vi "register update callback.vi"(8 "error in":errorcluster, 9 "controls":refnum<vi>[](array[refnum]), 10 "VI Refnum":refnum<vi>, 11 "displayable in":refnum<class "displayable.lvclass">) -> (0 "error out":errorcluster, 3 "displayable out":refnum<class "displayable.lvclass">)   [LabVIEW 2013, in "displayable.lvclass"]
uses:
  displayable.lvclass
  displayable.lvclass/displayable.ctl
  callback settings.ctl
  <vilib>/Utility/VariantDataType/VariantType.lvlib
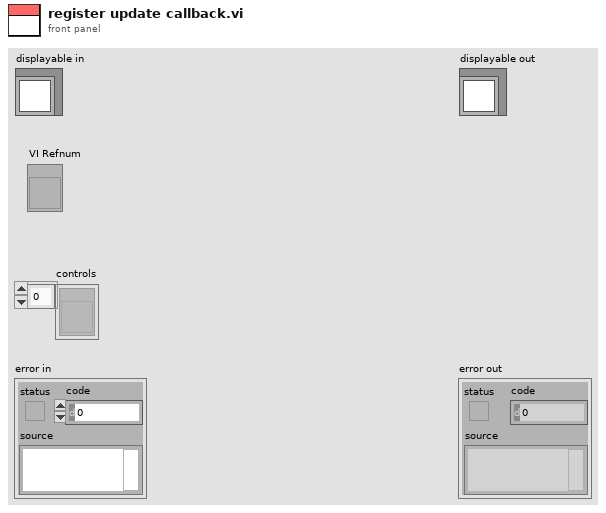
[diagram p1: front panel]
types:
  T1 = typedef "displayable.lvclass/callback settings.ctl" = cluster{"VI Refnum":refnum<vi>, "displayable":refnum<data-value>, "oi":string, "oo":string, "di":string}
  T2 = typedef "VariantType.lvlib/Type.ctl" = enum8{"Invalid Type", "Void", "I8", "I16", "I32", "I64", "U8", "U16", "U32", "U64", "Single Float", "Double Float", "Extended Float", "Single Complex", "Double Complex", "Extended Complex", "Enum U8", "Enum U16", "Enum U32", "Enum U64", "Single Float With Unit", "Double Float With Unit", "Extended Float With Unit", "Single Complex with Unit", "Double Complex with Unit", "Extended Complex with Unit", "Boolean", "String", "Path", "Picture", "Tag", "Array", "Cluster", "Variant", "LV Variant", "Waveform", "Timestamp", "Digital Waveform", "Digital Data", "ExpressData", "Refnum", "External Data", "VI", "Poly VI", "LabVIEW Class Instance", "Fixed Point"}
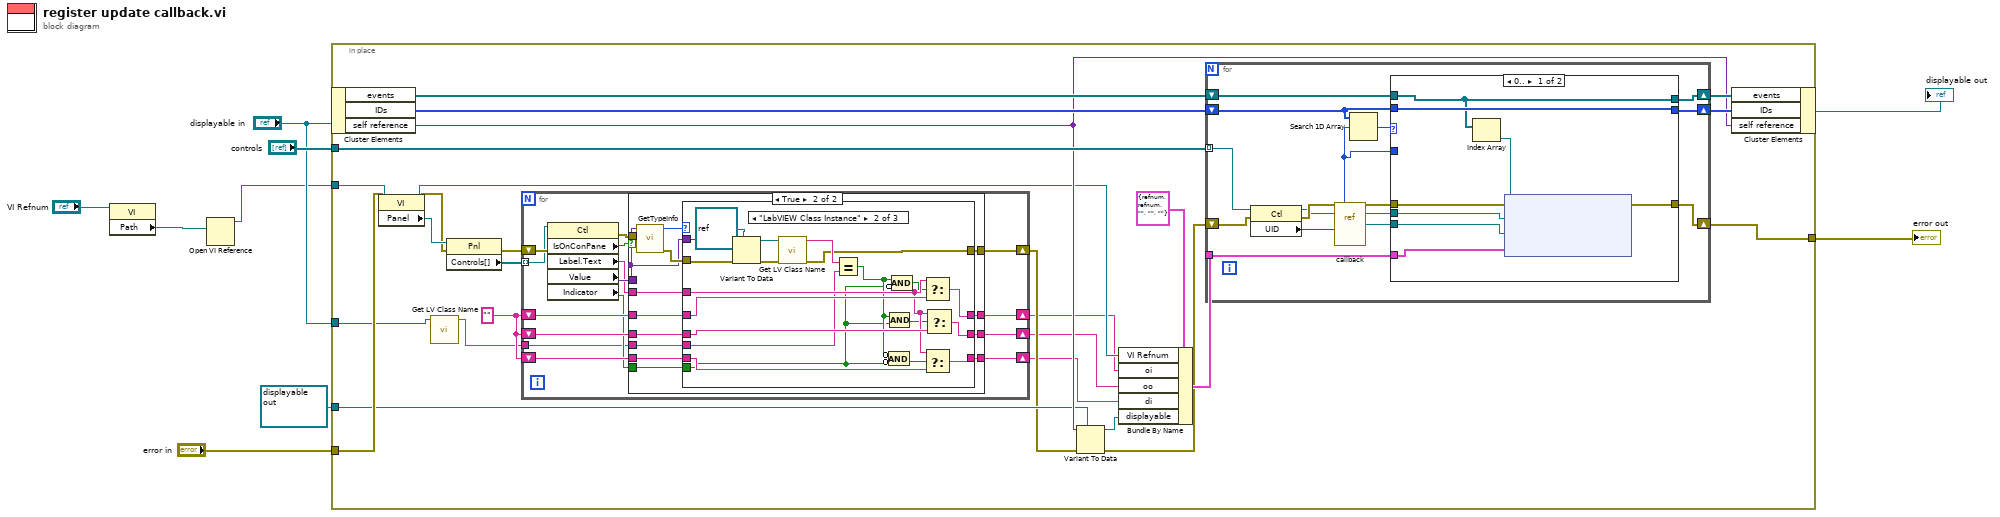
[diagram p0: block diagram]
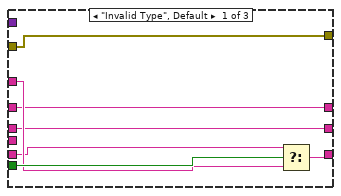
[diagram p3: hidden frame]
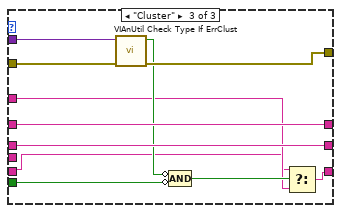
[diagram p4: hidden frame]
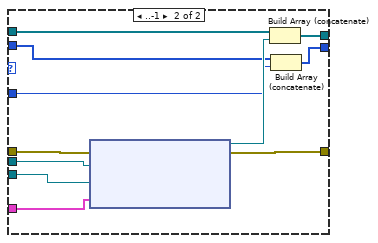
[diagram p5: hidden frame]
diagram:
  n1 = property class="VI"(reference="VI Refnum") -> ("Path"=w2:path)  [unwired: 1 in, 2 out]
  n2 = Open VI Reference(vi path=w2) -> (vi reference=w1:refnum<vi>)  [unwired: 5 in, 1 out]
  n3 = in-place {
    in-place-border: "controls" -> [w35]
    in-place-border: "error in" -> [w23]
    in-place-border: [w30] -> w6
    in-place-border: w1 -> [w27]
    in-place-border: refnum<data-value> refnum ("displayable") -> [w19]
    in-place-border: "displayable in" -> [w11]
    w15 = ""
    n4 = in-place-cluster #1("displayable in") -> ("events"=w34:refnum<k27>[], "IDs"=w33:i32[], "self reference"=w25:variant)
    n5 = property class="VI"(reference=w27, error in=w23) -> (reference out=w24:refnum<vi>, error out=w21:errorcluster, "Panel"=w22:refnum<vi>)
    n6 = call <vilib>:"Get LV Class Name.vi"("object"=w11) -> ("class name"=w10:string)  [unwired: 9 in, 1 out]
    n7 = property class="Pnl"(reference=w22, error in=w21) -> (error out=w17:errorcluster, "Controls[]"=w18:refnum<vi>[])  [unwired: 1 out]
    n8 = for {
      tunnel: w18 -> [w49] mode=indexing
      shift-right: [w46] -> w16
      shift-left: w17 -> [w50]
      shift-right: [w43] -> w14
      shift-left: w15 -> [w44]
      shift-right: [w42] -> w12
      shift-left: w15 -> [w41]
      shift-right: [w39] -> w13
      shift-left: w15 -> [w40]
      tunnel: w10 -> [w36]
      n9 = property class="Ctl"(reference=w49, error in=w50) -> (error out=w48:errorcluster, "IsOnConPane"=w45:bool, "Label.Text"=w37:string, "Value"=w47:variant, "Indicator"=w38:bool)  [unwired: 1 out]
      n10 = case shown="True" w45 {
        tunnel: w48 -> [w54 w68]
        tunnel: w47 -> [_ w65]
        tunnel: [w54 w64] -> w46
        tunnel: w44 -> [w53 w62]
        tunnel: [w53 w63] -> w43
        tunnel: [w52 w61] -> w42
        tunnel: w41 -> [w52 w60]
        tunnel: w40 -> [w51 w59]
        tunnel: [w51 w56] -> w39
        tunnel: w38 -> [_ w58]
        tunnel: w37 -> [_ w57]
        tunnel: w36 -> [_ w55]
        frame False {
        }
        frame True {
          n11 = call <vilib>:"GetTypeInfo.vi"("error in (no error)"=w68, "Variant"=w65) -> ("error out"=w66:errorcluster, "Type Enum"=w67:T2)  [unwired: 5 in, 3 out]
          n12 = case shown="\"LabVIEW Class Instance\"" w67 {
            tunnel: w66 -> [w69 w82 w106]
            tunnel: w65 -> [_ w81 w105]
            tunnel: [w69 w77 w104] -> w64
            tunnel: [w70 w95 w103] -> w63
            tunnel: w62 -> [w70 w90 w103]
            tunnel: [w71 w93 w102] -> w61
            tunnel: w60 -> [w71 w91 w102]
            tunnel: w59 -> [w73 w92 w97]
            tunnel: w58 -> [w75 w83 w100]
            tunnel: w57 -> [w74 w89 w98]
            tunnel: [w72 w94 w96] -> w56
            tunnel: w55 -> [_ w88 _]
            frame "Invalid Type", Default {
              n13 = Select(t=w73, s=w75, f=w74) -> (s? t:f=w72:string)
            }
            frame "LabVIEW Class Instance" {
              n14 = Variant To Data(error in=w82, type=refnum<class> refnum ("LabVIEW Object"), Variant=w81) -> (data=w79:refnum<class>, error out=w80:errorcluster)
              n15 = call <vilib>:"Get LV Class Name.vi"("error in (no error)"=w80, "object"=w79) -> ("error out"=w77:errorcluster, "class name"=w78:string)  [unwired: 8 in]
              n16 = Equal?(x=w78, y=w88) -> (x = y?=w84:bool)
              n17 = Compound Arithmetic op=AND(invert w84, invert w83) -> (w85:bool)
              n18 = Compound Arithmetic op=AND(w84, w83) -> (w87:bool)
              n19 = Compound Arithmetic op=AND(w84, invert w83) -> (w86:bool)
              n20 = Select(t=w89, s=w86, f=w90) -> (s? t:f=w95:string)
              n21 = Select(t=w89, s=w85, f=w92) -> (s? t:f=w94:string)
              n22 = Select(t=w89, s=w87, f=w91) -> (s? t:f=w93:string)
            }
            frame "Cluster" {
              n23 = call <vilib>:"VIAnUtil Check Type If ErrClust.vi"("error in (no error)"=w106, "Data In"=w105) -> ("error out"=w104:errorcluster, "IsErrClust?"=w101:bool)  [unwired: 8 out]
              n24 = Compound Arithmetic op=AND(invert w101, invert w100) -> (w99:bool)
              n25 = Select(t=w97, s=w99, f=w98) -> (s? t:f=w96:string)
            }
          }
        }
      }
    }
    n26 = Variant To Data(error in=w16, type=w19, Variant=w25) -> (data=w20:refnum<data-value>, error out=w26:errorcluster)
    n27 = Bundle By Name(cluster=T1 {"VI Refnum"=refnum, "displayable"=refnum, "oi"="", "oo"="", "di"=""} ("callback settings"), "VI Refnum"=w24, "oi"=w14, "oo"=w12, "di"=w13, "displayable"=w20) -> (w28:T1)
    n28 = for {
      tunnel: w35 -> [w119] mode=indexing
      shift-right: [w113] -> w31
      shift-left: w33 -> [w111]
      shift-right: [w112] -> w32
      shift-left: w34 -> [w114]
      shift-right: [w116] -> w30
      shift-left: w26 -> [w118]
      tunnel: w28 -> [w108]
      n29 = property class="Ctl"(reference=w119, error in=w118) -> (reference out=w109:refnum<vi>, error out=w117:errorcluster, "UID"=w110:i32)
      n30 = vi-ref "callback.vi"() -> ("vi reference"=w107:refnum<vi>)
      n31 = Search 1D Array(1D array=w111, element=w110) -> (index of element=w115:i32)  [unwired: 1 in]
      n32 = case shown="0.." w115 {
        tunnel: w117 -> [w125 w138]
        tunnel: [w123 w137] -> w116
        tunnel: w114 -> [w126 w136]
        tunnel: [w127 w134] -> w113
        tunnel: [w126 w133] -> w112
        tunnel: w111 -> [w127 w132]
        tunnel: w110 -> [_ w131]
        tunnel: w109 -> [w121 w130]
        tunnel: w108 -> [w120 w129]
        tunnel: w107 -> [w122 w128]
        frame 0.. {
          n33 = Index Array(array=w126) -> (element=w124:refnum<k27>)  [unwired: 1 in]
          n34 = node(w124, w125, w121, w122, w120) -> (w123:errorcluster)  [unwired: 1 out]
        }
        frame ..-1 {
          n35 = node(w138, w130, w128, w129) -> (w135:refnum<k27>, w137:errorcluster)  [unwired: 1 in]
          n36 = Build Array (concatenate)(w136, w135) -> (w133:refnum<k27>[])
          n37 = Build Array (concatenate)(w132, w131) -> (w134:i32[])
        }
      }
    }
    n38 = in-place-cluster #1("events"=w32, "IDs"=w31, "self reference"=w25) -> (→"displayable out":refnum<class "displayable.lvclass">)
  }
  "error out" <- w6
